vi "pump rpm 3-stop color code.vi"(0 "flow rate":dbl[unit] format="%.2f", 1 "3-stop tubing":T1) -> (3 "pump speed (rpm)":dbl format="%.2f", 5 "in range":bool)   [LabVIEW 2010]
uses:
  Stamp/calibration commands.ctl
  3-stop colors.ctl
panel:
  in  "IDs":sgl[](array[numeric])=[0.13, 0.19, 0.25, 0.38, 0.44, 0.51, 0.57, 0.64, 0.76, 0.89, 0.95, 1.02, 1.09, 1.14, 1.22, 1.3, 1.42, 1.52, 1.65, 1.75, 1.85, 2.06, 2.29, 2.54, 2.79, 3.17, 0.79375, 1.5875, 4.8, 3.175, 6.35, 7.9375] format="%.3f"
  # "orange-black\norange-red\norange-blue\norange-green\ngreen-yellow\norange-yellow\nwhite-yellow\norange-white\nblack-black\norange-orange\nwhite-black\nwhite-white\nwhite-red\nred-red\nred-grey\ngrey-grey\nyellow-yellow\nyellow-blue\nblue-blue\nblue-green\ngreen-green\npurple-purple\npurple-black\npurple-orange\npurple-white\nblack-white\n13\n14\n15\n16\n17\n18"
  # "13"
  # "14"
  # "15"
  # "16"
  # "17"
  # "18"
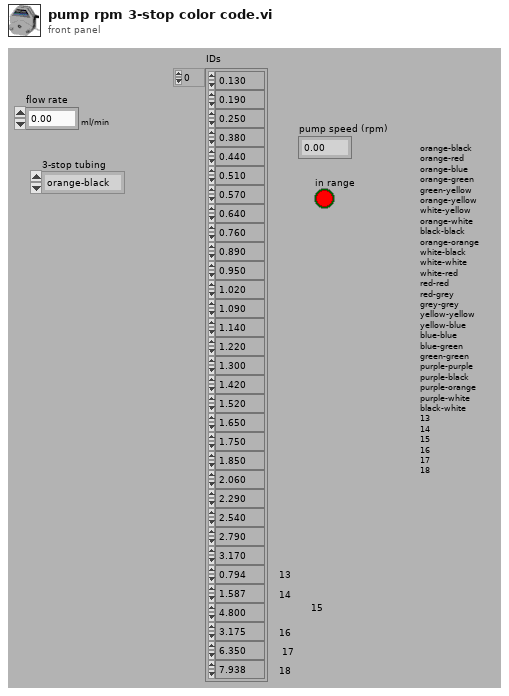
[diagram p1: front panel]
types:
  T1 = typedef "3-stop colors.ctl" = enum16{"orange-black", "orange-red", "orange-blue", "orange-green", "green-yellow", "orange-yellow", "white-yellow", "orange-white", "black-black", "orange-orange", "white-black", "white-white", "white-red", "red-red", "red-grey", "grey-grey", "yellow-yellow", "yellow-blue", "blue-blue", "blue-green", "green-green", "purple-purple", "purple-black", "purple-orange", "purple-white", "black-white", "13", "14", "15", "16", "17", "18"}
  T2 = typedef "calibration commands.ctl" = enum16{"Get ini Path", "Save default values", "Save new calibration", "Read calibration", "Apply calibration", "Read STAMP mb", "Write STAMP mb"}
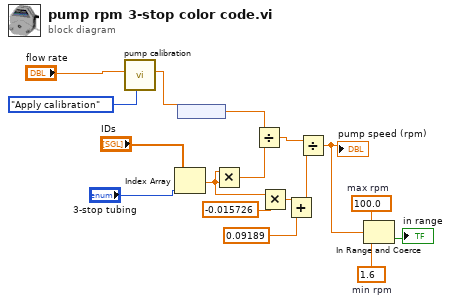
[diagram p0: block diagram]
diagram:
  w9 = 1.6  # min rpm
  w10 = 100.0  # max rpm
  n1 = call "pump calibration.vi"("pump cal command"=calibration_commands."Apply calibration", "flow rate"="flow rate") -> ("modified flow rate"=w1:dbl[unit])  [unwired: 3 in, 3 out]
  n2 = Index Array(array="IDs", index="3-stop tubing") -> (element=w4:sgl)
  n3 = node(w1) -> (w16:dbl)
  n4 = Multiply(x=w4, y=w4) -> (x*y=w7:sgl)
  n5 = Divide(x=w16, y=w7) -> (x/y=w15:dbl)
  n6 = Multiply(x=w4, y=-0.015726) -> (x*y=w13:dbl)
  n7 = Add(x=w13, y=0.09189) -> (x+y=w11:dbl)
  n8 = Divide(x=w15, y=w11) -> (x/y=w8:dbl)
  "pump speed (rpm)" <- w8
  n9 = In Range and Coerce(upper limit=w10, x=w8, lower limit=w9) -> (In Range?=→"in range":bool)  [unwired: 1 out]
